vi "YAML_bool.vi"(1 "value":bool=TRUE, 2 "name":string) -> (0 "result":string)   [LabVIEW 2011]
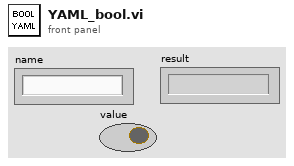
[diagram p1: front panel]
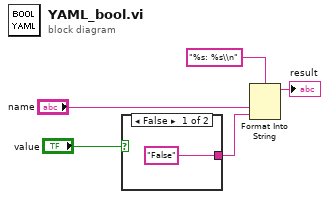
[diagram p0: block diagram]
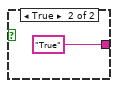
[diagram p2: hidden frame]
diagram:
  n1 = case shown="False" "value" {
    tunnel: ["False" ("format string") "True" ("format string")] -> w1
    frame False {
    }
    frame True {
    }
  }
  n2 = Format Into String(format string="%s: %s\\n", "name", w1) -> (resulting string=→"result":string)  [unwired: 2 in, 1 out]
